vi "Gergberg Image Manipulation.vi"() -> ()   [LabVIEW 2012, in "LightPipes.lvlib"]
uses:
  LightPipes.lvlib
  <vilib>/vision/NI_Vision_Development_Module.lvlib
panel:
  in  "MF Rotate 180":bool=TRUE
  in  "Balance Energy":bool=TRUE
  out "FF Interp Size":cluster{"x":i32, "y":i32}={"x"=1000, "y"=1000}
  out "FF Interp Pic":T1(plugin-control)
  in  "FF Crop Size":i32=400
  in  "FF Interp Ratio":dbl=2.5
  in  "Far Field":path=path "C:/Users/Tri Nguyen/Downloads/MidfieldFarfieldForAaron/MidfieldFarfieldForAaron/005778 2013-02-12/Masked FF.png"
  in  "MF Crop Size":i32=1000
  out "MF Interp Size":cluster{"x":i32, "y":i32}={"x"=1000, "y"=1000}
  out "MF Interped Pic":T1(plugin-control)
  in  "MF Interp Ratio":dbl=1.0
  in  "Mid Field":path=path "C:/Users/Tri Nguyen/Downloads/MidfieldFarfieldForAaron/MidfieldFarfieldForAaron/005778 2013-02-12/Masked MF.png"
  # "1. Balance Energy: normalize MF and FF energy to the same. MF is used as the base\n2. MF Rotate 180: will rotate MF image 180 degree"
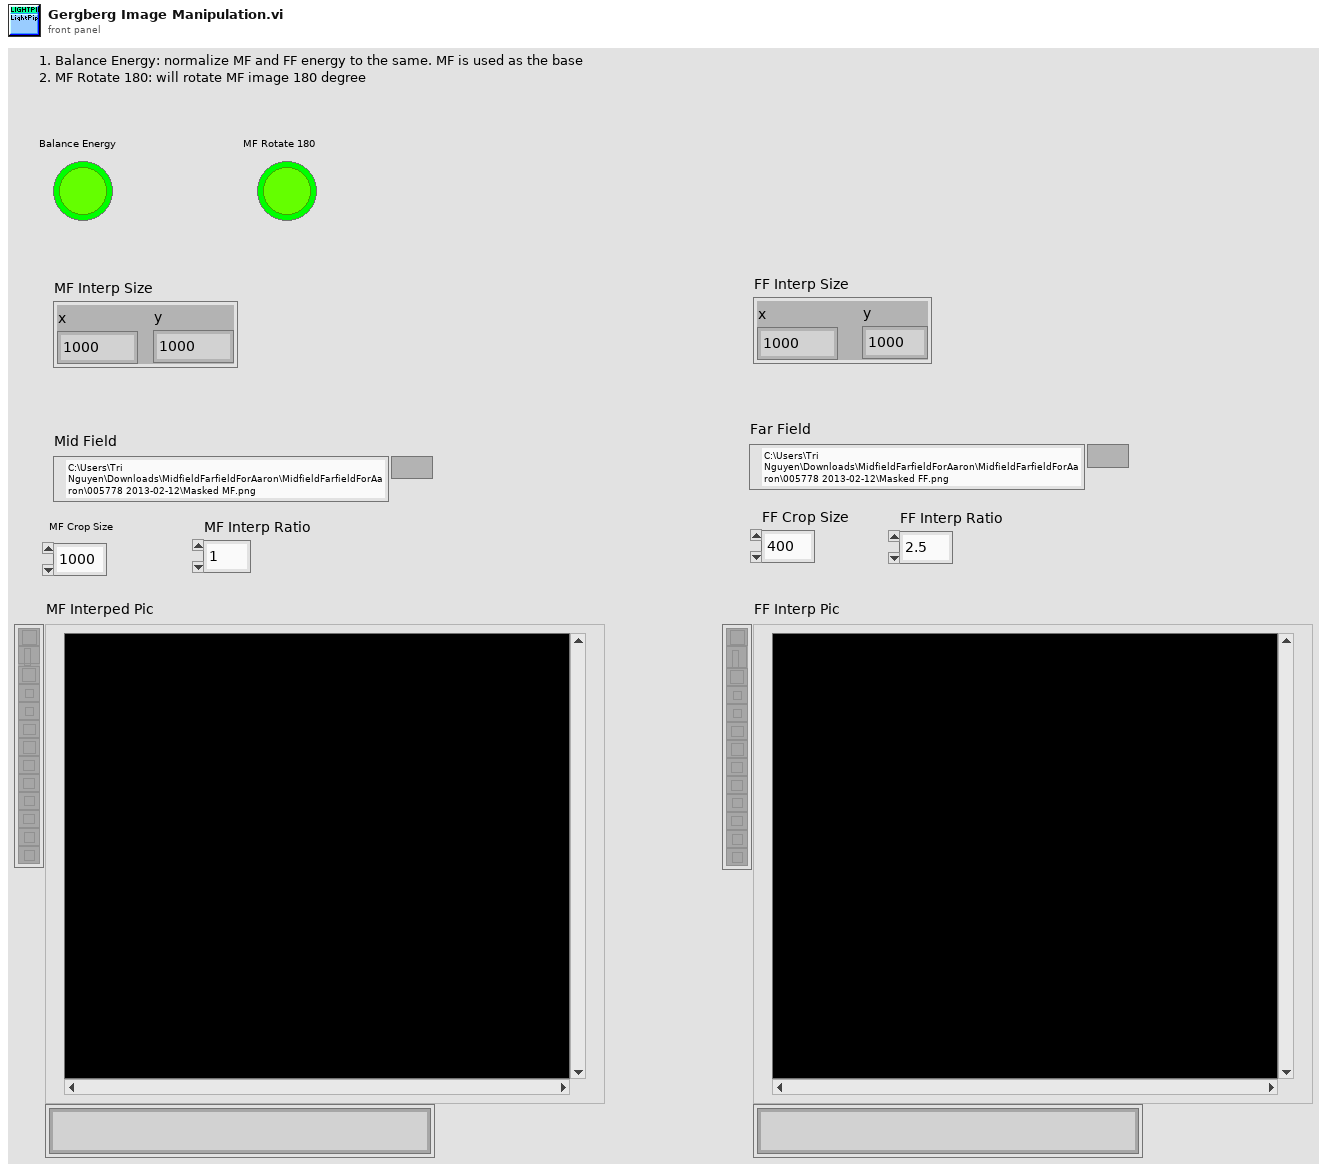
[diagram p1: front panel]
types:
  T1 = typedef "IMAQ Image.ctl" = refnum<image>
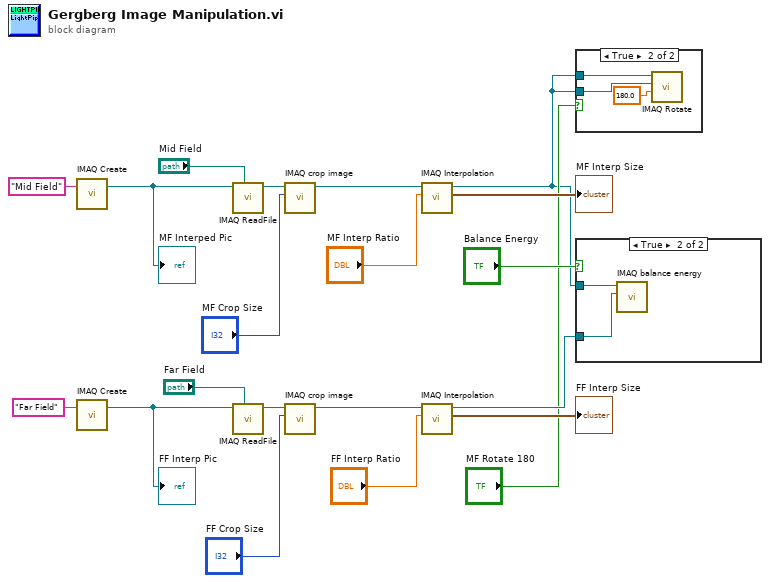
[diagram p0: block diagram]
diagram:
  n1 = call "IMAQ Create"("Image Name"="Mid Field") -> ("New Image"=w10:T1)  [unwired: 4 in, 1 out]
  "MF Interped Pic" <- w10
  n2 = call "IMAQ Create"("Image Name"="Far Field") -> ("New Image"=w9:T1)  [unwired: 4 in, 1 out]
  "FF Interp Pic" <- w9
  n3 = call "IMAQ ReadFile"("File Path"="Mid Field", "Image"=w10) -> ("Image Out"=w12:T1)  [unwired: 3 in, 6 out]
  n4 = call "IMAQ ReadFile"("File Path"="Far Field", "Image"=w9) -> ("Image Out"=w5:T1)  [unwired: 3 in, 6 out]
  n5 = call "IMAQ crop image.vi"("Image"=w12, "Square Image Size"="MF Crop Size") -> ("Cropped"=w17:T1)  [unwired: 8 in]
  n6 = call "IMAQ crop image.vi"("Image"=w5, "Square Image Size"="FF Crop Size") -> ("Cropped"=w7:T1)  [unwired: 8 in]
  n7 = call "IMAQ Interpolation.vi"("Ratio"="MF Interp Ratio", "Image In"=w17) -> ("Interpolated Image Size"=→"MF Interp Size":cluster{"x":i32, "y":i32}, "Interpolated Image"=w1:T1)  [unwired: 8 in]
  n8 = call "IMAQ Interpolation.vi"("Ratio"="FF Interp Ratio", "Image In"=w7) -> ("Interpolated Image Size"=→"FF Interp Size":cluster{"x":i32, "y":i32}, "Interpolated Image"=w3:T1)  [unwired: 8 in]
  n9 = case shown="True" "MF Rotate 180" {
    tunnel: w1 -> [_ w22]
    tunnel: w1 -> [_ w21]
    frame False {
    }
    frame True {
      n10 = call "IMAQ Rotate"("Angle (degrees)"=sgl 180.0, "Image Dst"=w21, "Image Src"=w22) -> ()  [unwired: 7 in, 2 out]
    }
  }
  n11 = case shown="True" "Balance Energy" {
    tunnel: w1 -> [_ w25]
    tunnel: w3 -> [_ w24]
    frame False {
    }
    frame True {
      n12 = call "IMAQ balance energy.vi"("Target Image"=w24, "Base Image"=w25) -> ()  [unwired: 9 in, 1 out]
    }
  }
